vi "NoParent_TreeHasTagWithPrefixAndName.vi"() -> (0 "error out":errorcluster)   [LabVIEW 2017, in "ResultTree.Tests.lvlib" / "AddTestCase.lvlib"]
uses:
  AddTestCase.lvlib
  883aa515-c0c6-4eeb-ba88-1d0faa620524.vi
  Constraint/IsEqual/Create.vi
  Constraint/IsEqual/IsEqual.lvclass
  ResultTree/ResultTree.lvclass
panel:
  in  "Tree":string(tree)
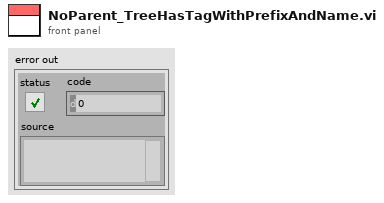
[diagram p1: front panel]
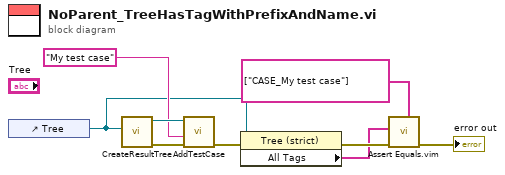
[diagram p0: block diagram]
diagram:
  n1 = control-ref of="Tree"() -> (w1:refnum<vi>)
  n2 = call "CreateResultTree.vi"("Tree Refnum"=w1) -> ("error out"=w9:errorcluster, "ResultTree out"=w8:refnum<class "ResultTree.lvclass">)  [unwired: 9 in]
  n3 = call "AddTestCase.vi"("error in (no error)"=w9, "Name"="My test case", "ResultTree in"=w8) -> ("error out"=w3:errorcluster)  [unwired: 6 in, 2 out]
  n4 = property class="Tree (strict)"(reference=w1, error in=w3) -> (error out=w6:errorcluster, "All Tags"=w5:string[])  [unwired: 1 out]
  n5 = call "Assert Equals.vim"("Expected"=string[] ["CASE_My test case"] ("All Tags"), "error in (no error)"=w6, "Actual"=w5) -> ("error out"=→"error out":errorcluster)  [unwired: 8 in]
